vi "Write Ch Select.vi"(8 "error in (no error)":errorcluster, 10 "Ch Select":i32[](array[numeric]), 11 "Lakeshore 325 in":refnum<class "Lakeshore 325.lvclass">) -> (0 "error out":errorcluster, 3 "Lakeshore 325 out":refnum<class "Lakeshore 325.lvclass">)   [LabVIEW 2022 SP3, in "Lakeshore 325.lvclass"]
uses:
  Lakeshore 325.lvclass
  Lakeshore 325.lvclass/Lakeshore 325.ctl
  Temp Control.lvclass
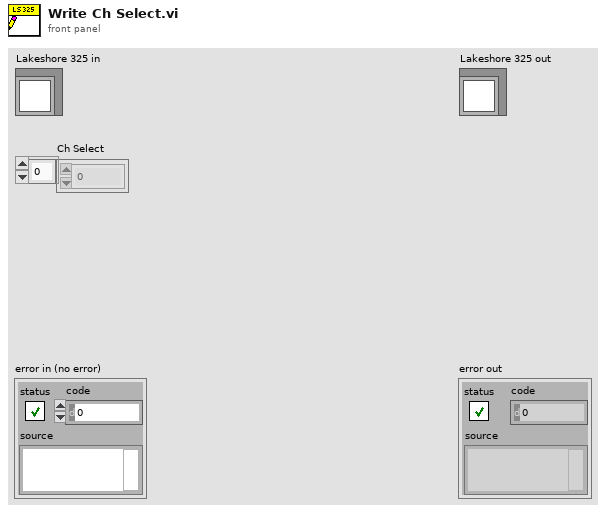
[diagram p1: front panel]
types:
  T1 = typedef "Lakeshore 325.lvclass/Lakeshore 325 Settings cluster.ctl" = cluster{"Addr":refnum<visa-resource-name>, "Ch Prefix":string, "Ch Select":i32[]}
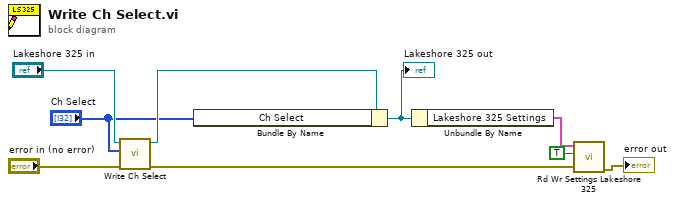
[diagram p0: block diagram]
diagram:
  n1 = call-parent "Write Ch Select.vi"("error in (no error)"="error in (no error)", "Ch Select"="Ch Select", "Temp Control in"="Lakeshore 325 in") -> ("error out"=w2:errorcluster, "Temp Control out"=w7:refnum<class "Lakeshore 325.lvclass">)  [unwired: 7 in]
  n2 = Bundle By Name(cluster=w7, "Ch Select"="Ch Select") -> (w5:refnum<class "Lakeshore 325.lvclass">)
  "Lakeshore 325 out" <- w5
  n3 = Unbundle By Name(w5) -> ("Lakeshore 325 Settings"=w4:T1)
  n4 = call "Rd Wr Settings Lakeshore 325.vi"("error in (no error)"=w2, "Write? (F:Read)"=TRUE, "Lakeshore 325 Settings"=w4) -> ("error out"=→"error out":errorcluster)  [unwired: 7 in, 1 out]
